vi "control_part_number.vi"(7 "select_for_part_number":T1, 10 "find_part":string, 11 "parts_number":string[][](array[string])) -> (2 "find_type_part?":bool, 3 "finded_part_number":string)   [LabVIEW 2020]
uses:
  control_part_number.ctl
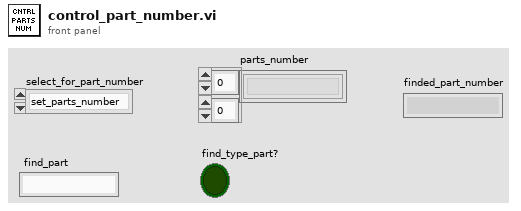
[diagram p1: front panel]
types:
  T1 = typedef "control_part_number.ctl" = enum16{"set_parts_number", "get_part_number_by_name"}
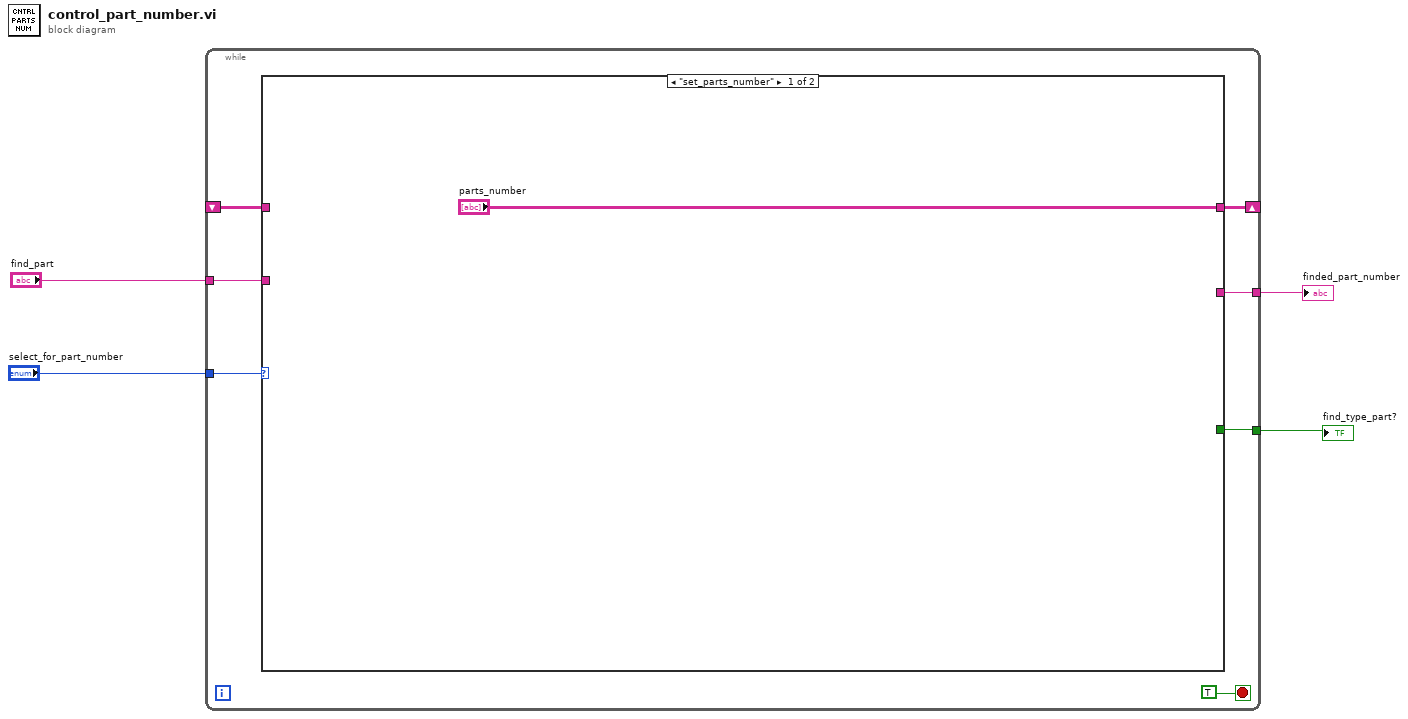
[diagram p0: block diagram]
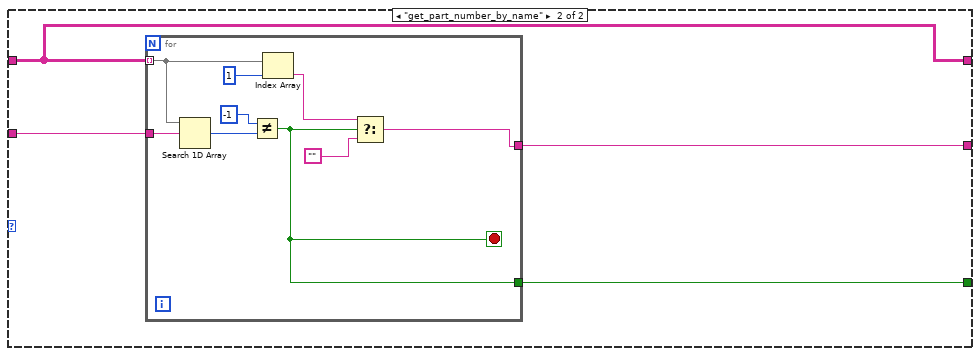
[diagram p2: hidden frame]
diagram:
  n1 = while {
    tunnel: "select_for_part_number" -> [w10]
    shift-right: [w8] -> _
    shift-left: _ -> [w7]
    tunnel: "find_part" -> [w9]
    tunnel: [w6] -> w2
    tunnel: [w5] -> w1
    stop <- TRUE stop-if-true
    n2 = case shown="\"set_parts_number\"" w10 {
      tunnel: w9 -> [_ w16]
      tunnel: ["parts_number" w15] -> w8
      tunnel: w7 -> [_ w15]
      tunnel: [_ w14] -> w6
      tunnel: [_ w13] -> w5
      frame "set_parts_number" {
      }
      frame "get_part_number_by_name" {
        n3 = for {
          tunnel: w15 -> [w21] mode=indexing
          tunnel: w16 -> [w25]
          tunnel: [w17] -> w14
          tunnel: [w22] -> w13
          stop <- w22 stop-if-true
          n4 = Search 1D Array(1D array=w21, element=w25) -> (index of element=w24:i32)  [unwired: 1 in]
          n5 = Not Equal?(x=-1, y=w24) -> (x != y?=w22:bool)
          n6 = Index Array(array=w21, index=1) -> (element=w19:string)
          n7 = Select(t=w19, s=w22, f="") -> (s? t:f=w17:string)
        }
      }
    }
  }
  "finded_part_number" <- w2
  "find_type_part?" <- w1
